vi "get_unit_vector.vi"(8 "error in (no error)":errorcluster, 11 "SpaceVector in":refnum<class "SpaceVector.lvclass">) -> (0 "error out":errorcluster, 2 "unit vector":refnum<class "SpaceVector.lvclass">, 3 "SpaceVector out":refnum<class "SpaceVector.lvclass">)   [LabVIEW 2010, in "SpaceVector.lvclass"]
uses:
  SpaceVector.lvclass
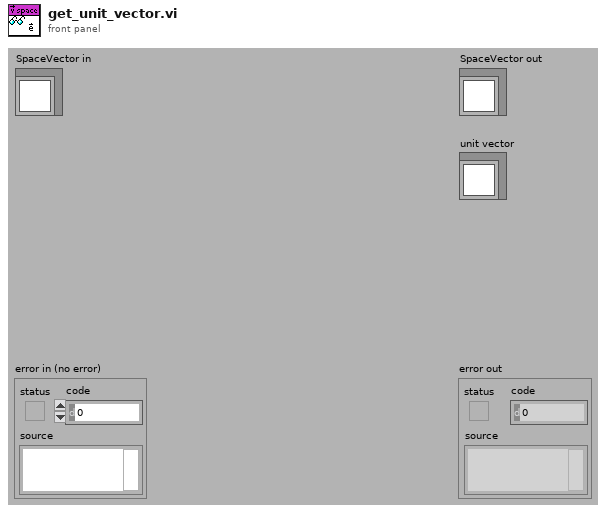
[diagram p1: front panel]
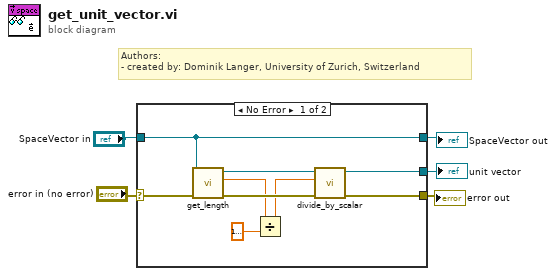
[diagram p0: block diagram]
diagram:
  # "Authors: \n- created by: Dominik Langer, University of Zurich, Switzerland"
  n1 = case shown="No Error" "error in (no error)" {
    selector: "error in (no error)" -> [w11 w16]
    tunnel: [w10 w16] -> w4
    tunnel: [w14 w15] -> w2
    tunnel: "SpaceVector in" -> [w14 w15]
    tunnel: [w9 _] -> w1
    frame No Error {
      n2 = call "get_length.vi"("error in (no error)"=w11, "SpaceVector in"=w14) -> ("error out"=w12:errorcluster, "length"=w8:dbl[unit], "SpaceVector out"=w13:refnum<class "SpaceVector.lvclass">)  [unwired: 7 in]
      n3 = Divide(x=w8, y=dbl[unit] 1e-06) -> (x/y=w6:dbl)
      n4 = call "divide_by_scalar.vi"("error in (no error)"=w12, "divisor"=w6, "SpaceVector in"=w13) -> ("error out"=w10:errorcluster, "SpaceVector out"=w9:refnum<class "SpaceVector.lvclass">)  [unwired: 7 in]
    }
    frame Error {
    }
  }
  "error out" <- w4
  "SpaceVector out" <- w2
  "unit vector" <- w1
